vi "Switch Box Resistor Select Control.vi"(0 "PhyChls":tag="Dev1/port0/line5, Dev1/port0/line7, Dev1/port1/line0", 1 "line grouping":i32(ring) items=["one channel for each line", "one channel for all lines"], 2 "Resistor":T1(ring), 5 "All OFF":bool, 7 "Dout Inv":bool[](array[boolean])=[FALSE, FALSE, FALSE], 11 "ErrIn":errorcluster, 12 "SimOn":bool, 13 "Init":bool, 14 "Stop":bool) -> (15 "ErrOut":errorcluster)   [LabVIEW 2013]
uses:
  <vilib>/DAQmx/write.llb/DAQmx Write (Digital 1D Bool NChan 1Samp 1Line).vi
  <vilib>/DAQmx/create/channels.llb/DAQmx Create Channel (DO-Digital Output).vi
  <vilib>/DAQmx/miscellaneous.llb/DAQmx Fill In Error Info.vi
panel:
  out "Douts":bool[](array[boolean])
  # "ER2007"
  # "RSCL1 -> RSCL3"
  # "R1 - 10 ohm\nR2 - 100 ohm\nR3 - 1 Kohm\nR4 - 10 Kohm\nR5 - 100 Kohm\nR6 - 1 megohm"
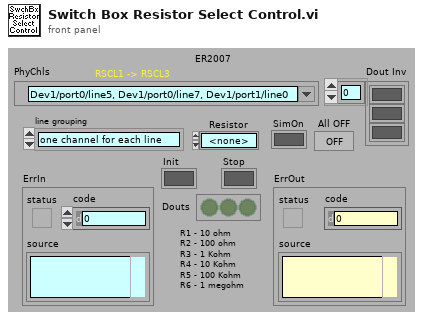
[diagram p1: front panel]
types:
  T1 = enum16{"<none>", "Resistor 1", "Resistor 2", "Resistor 3", "Resistor 4", "Resistor 5", "Resistor 6"}
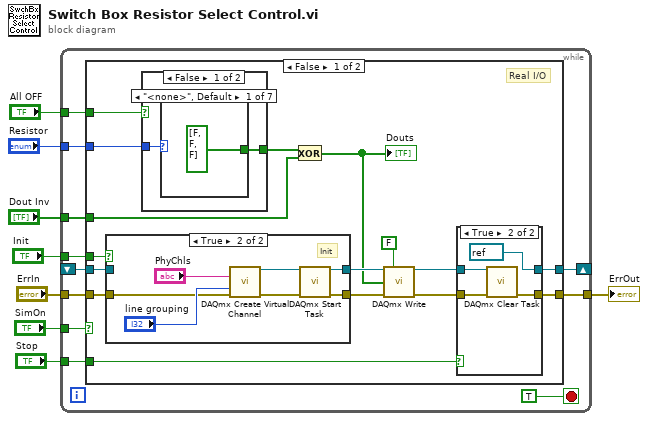
[diagram p0: block diagram]
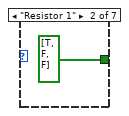
[diagram p4: hidden frame]
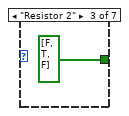
[diagram p5: hidden frame]
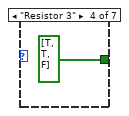
[diagram p6: hidden frame]
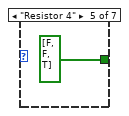
[diagram p7: hidden frame]
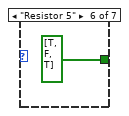
[diagram p8: hidden frame]
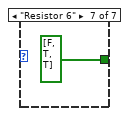
[diagram p9: hidden frame]
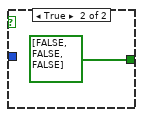
[diagram p10: hidden frame]
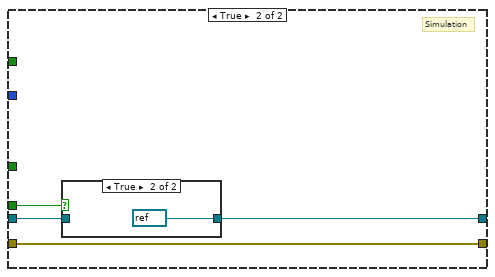
[diagram p11: hidden frame]
diagram:
  n1 = while {
    tunnel: "ErrIn" -> [w19]
    tunnel: [w18] -> w7
    tunnel: "SimOn" -> [w17]
    tunnel: "Stop" -> [w16]
    shift-right: [w14] -> _
    shift-left: _ -> [w13]
    tunnel: "All OFF" -> [w12]
    tunnel: "Resistor" -> [w11]
    tunnel: "Init" -> [w10]
    tunnel: "Dout Inv" -> [w9]
    stop <- TRUE stop-if-true
    n2 = case shown="False" w17 {
      tunnel: w19 -> [w35 w64]
      tunnel: [w29 w64] -> w18
      tunnel: w16 -> [w27 _]
      tunnel: [w26 w61] -> w14
      tunnel: w13 -> [w25 w62]
      tunnel: w12 -> [w24 _]
      tunnel: w11 -> [w23 _]
      tunnel: w10 -> [w22 w63]
      tunnel: w9 -> [w21 _]
      frame False {
        # "Real I/O"
        n3 = case shown="True" w22 {
          tunnel: w35 -> [w36 w42]
          tunnel: [w36 w40] -> w34
          tunnel: [w37 w38] -> w33
          tunnel: w25 -> [w37 _]
          frame False {
          }
          frame True {
            # "Init"
            n4 = call-poly <vilib>:"DAQmx Create Virtual Channel.vi"("lines"="PhyChls", "line grouping"="line grouping", "error in"=w42) -> ("task out"=w39:refnum<k21>, "error out"=w41:errorcluster)  [unwired: 11 in]
            n5 = call <vilib>:"DAQmx Start Task.vi"("task/channels in"=w39, "error in"=w41) -> ("task out"=w38:refnum<k21>, "error out"=w40:errorcluster)  [unwired: 12 in]
          }
        }
        n6 = case shown="False" w24 {
          tunnel: [w51 bool[] [FALSE, FALSE, FALSE]] -> w28
          tunnel: w23 -> [w52 _]
          frame False {
            n7 = case shown="\"<none>\", Default" w52 {
              tunnel: [bool[] [FALSE, FALSE, FALSE] bool[] [TRUE, FALSE, FALSE] bool[] [FALSE, TRUE, FALSE] bool[] [TRUE, TRUE, FALSE] bool[] [FALSE, FALSE, TRUE] bool[] [TRUE, FALSE, TRUE] bool[] [FALSE, TRUE, TRUE]] -> w51
              frame "<none>", Default {
              }
              frame "Resistor 1" {
              }
              frame "Resistor 2" {
              }
              frame "Resistor 3" {
              }
              frame "Resistor 4" {
              }
              frame "Resistor 5" {
              }
              frame "Resistor 6" {
              }
            }
          }
          frame True {
          }
        }
        n8 = Exclusive Or(1:w21, 2:w28) -> (0:w20:bool[])
        "Douts" <- w20
        n9 = call-poly <vilib>:"DAQmx Write.vi"("task/channels in"=w33, "auto start"=FALSE, "data"=w20, "error in"=w34) -> ("task out"=w30:refnum<k21>, "error out"=w31:errorcluster)  [unwired: 9 in, 1 out]
        n10 = case shown="True" w27 {
          tunnel: w31 -> [w45 w50]
          tunnel: w30 -> [w46 w49]
          tunnel: [w45 w48] -> w29
          tunnel: [w46 refnum<k21> refnum ("task out")] -> w26
          frame False {
          }
          frame True {
            n11 = call <vilib>:"DAQmx Clear Task.vi"("task in"=w49, "error in"=w50) -> ("error out"=w48:errorcluster)  [unwired: 13 in]
          }
        }
      }
      frame True {
        # "Simulation"
        n12 = case shown="True" w63 {
          tunnel: w62 -> [w65 _]
          tunnel: [w65 refnum<k21> refnum ("task out")] -> w61
          frame False {
          }
          frame True {
          }
        }
      }
    }
  }
  "ErrOut" <- w7
